vi "GyroAdjust.vi"(1 "Encoder Ticks per rev":dbl, 2 "Gyro Position":dbl, 3 "Setpoint In":dbl) -> (0 "Setpoint Out":dbl)   [LabVIEW 2014]
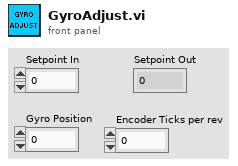
[diagram p1: front panel]
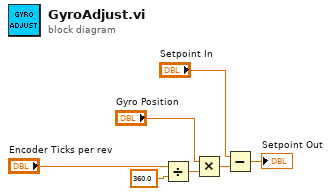
[diagram p0: block diagram]
diagram:
  n1 = Divide(x="Encoder Ticks per rev", y=360.0 ("x")) -> (x/y=w2:dbl)
  n2 = Multiply(x="Gyro Position", y=w2) -> (x*y=w4:dbl)
  n3 = Subtract(x="Setpoint In", y=w4) -> (x-y=→"Setpoint Out":dbl)
